vi "WPI_RobotDriveOpen2MotorWithSPARK.vi"(5 "Right Motor Inverted":bool, 7 "Left Motor Inverted":bool, 8 "error in (no error)":errorcluster, 10 "Right Motor":T4=enum."Invalid", 11 "Left Motor":T4=enum."Invalid") -> (0 "error out":errorcluster, 3 "RobotDriveDevRef":T1={"DevStatus"={"status"=FALSE, "code"=0, "source"=""}, "Motors[]"=[], "Square Inputs"=FALSE, "Max Output"=1.0})   [LabVIEW 2025]
doc: "Opens a reference to the robot drive for a two-motor robot using Rev Robotics SPARK motor controllers.\n\nThis software is licensed. Open the labview\\readme\\WPI Robotics Library Open Source License.txt file for more information."
uses:
  <vilib>/Rock Robotics/SystemInterfaces/DIO/FPGA_DIOPWMChannel.ctl
  <vilib>/Rock Robotics/WPI/RobotDrive/WPI_RobotDriveDevRef.ctl
  <vilib>/Rock Robotics/WPI/MotorControl/WPI_MotorControlDeviceRef.ctl
  <vilib>/Rock Robotics/WPI/MotorControl/WPI_MotorControlType.ctl
  <vilib>/Rock Robotics/WPI/PWM/WPI_PWMDeadband.ctl
  <vilib>/Rock Robotics/SystemInterfaces/DIO/FPGA_DIOChannel.ctl
  <vilib>/Rock Robotics/WPI/SafetyOutput/WPI_SafetyOutputConfigMenu.ctl
  <vilib>/Rock Robotics/WPI/MotorControl/WPI_MotorControlOpen SPARK.vi
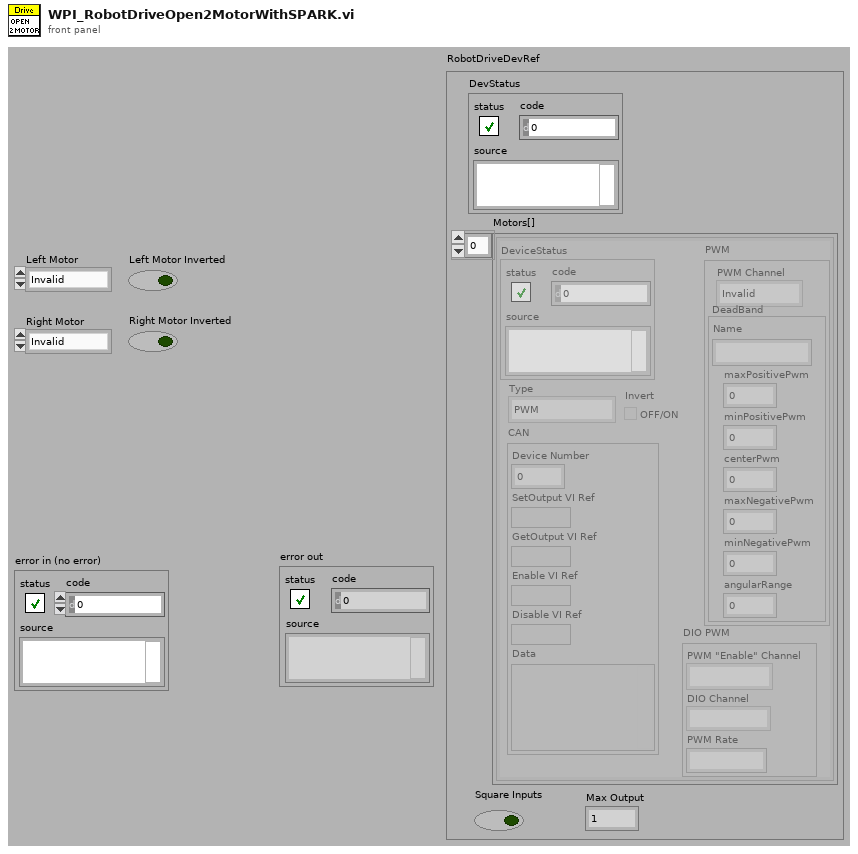
[diagram p1: front panel]
types:
  T1 = typedef "WPI_RobotDriveDevRef.ctl" = cluster{"DevStatus":errorcluster, "Motors[]":T2[], "Square Inputs":bool, "Max Output":dbl}
  T2 = typedef "WPI_MotorControlDeviceRef.ctl" = cluster{"DeviceStatus":errorcluster, "Type":T3, "PWM":cluster{"PWM Channel":T4, "DeadBand":T5}, "CAN":cluster{"Device Number":u8, "SetOutput VI Ref":variant, "GetOutput VI Ref":variant, "Enable VI Ref":variant, "Disable VI Ref":variant, "Data":variant}, "Invert":bool, "DIO PWM":cluster{"PWM \"Enable\" Channel":T4, "DIOChannel":T6, "PWM Rate":dbl}}
  T3 = typedef "WPI_MotorControlType.ctl" = enum16{"PWM", "CAN", "DIO PWM"}
  T4 = typedef "FPGA_DIOPWMChannel.ctl" = enum8{"PWM 0", "PWM 1", "PWM 2", "PWM 3", "PWM 4", "PWM 5", "PWM 6", "PWM 7", "PWM 8", "PWM 9", "PWM MXP 0", "PWM MXP 1", "PWM MXP 2", "PWM MXP 3", "PWM MXP 4", "PWM MXP 5", "PWM MXP 6", "PWM MXP 7", "PWM MXP 8", "PWM MXP 9", "Invalid"}
  T5 = typedef "WPI_PWMDeadband.ctl" = cluster{"Name":string, "maxPositivePwm":i32, "minPositivePwm":i32, "centerPwm":i32, "maxNegativePwm":i32, "minNegativePwm":i32, "angularRange":u16}
  T6 = typedef "FPGA_DIOChannel.ctl" = enum8{"DIO 0", "DIO 1", "DIO 2", "DIO 3", "DIO 4", "DIO 5", "DIO 6", "DIO 7", "DIO 8", "DIO 9", "DIO MXP 0", "DIO MXP 1", "DIO MXP 2", "DIO MXP 3", "DIO MXP 4", "DIO MXP 5", "DIO MXP 6", "DIO MXP 7", "DIO MXP 8", "DIO MXP 9", "DIO MXP 10", "DIO MXP 11", "DIO MXP 12", "DIO MXP 13", "DIO MXP 14", "DIO MXP 15", "SPI Port CS1", "SPI Port CS2", "SPI Port CS3", "SPI Port MISO", "SPI Port MOSI", "Invalid"}
  T7 = typedef "WPI_SafetyOutputConfigMenu.ctl" = enum16{"Enable", "Disable"}
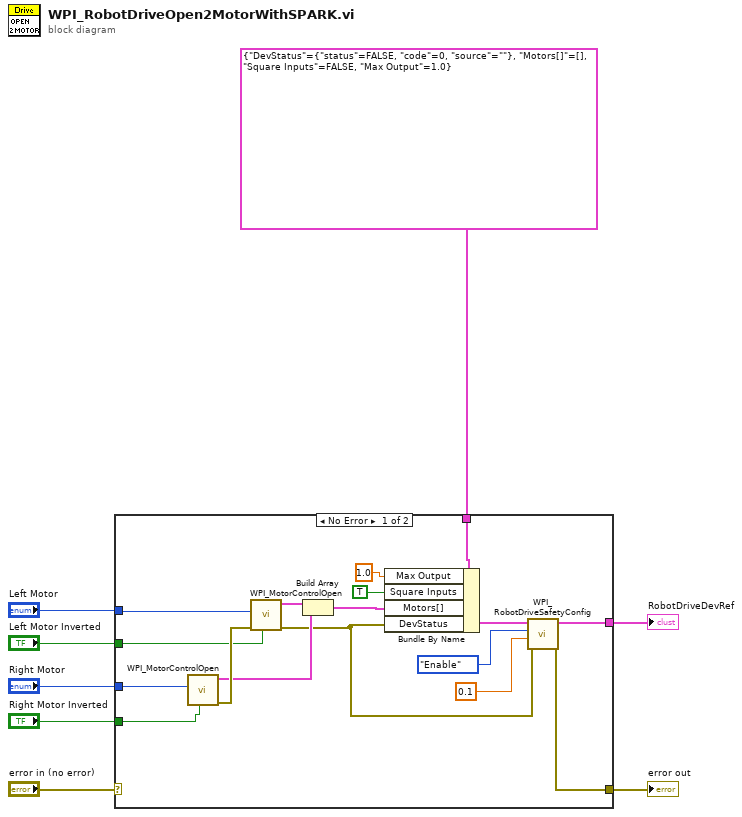
[diagram p0: block diagram]
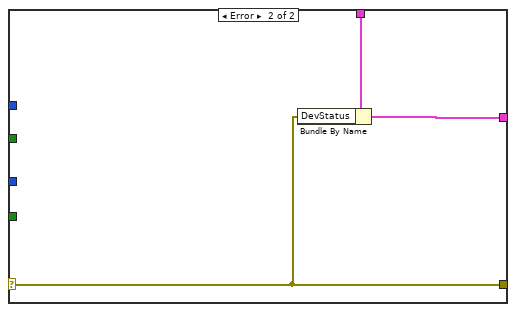
[diagram p2: hidden frame]
diagram:
  n1 = case shown="No Error" "error in (no error)" {
    selector: "error in (no error)" -> [_ w26]
    tunnel: "Left Motor" -> [w23 _]
    tunnel: "Right Motor" -> [w22 _]
    tunnel: [w11 w28] -> w1
    tunnel: "Left Motor Inverted" -> [w17 _]
    tunnel: "Right Motor Inverted" -> [w18 _]
    tunnel: T1 {"DevStatus"={"status"=FALSE, "code"=0, "source"=""}, "Motors[]"=[], "Square Inputs"=FALSE, "Max Output"=1.0} ("RobotDriveDevRef") -> [w24 w27]
    tunnel: [w12 w26] -> w3
    frame No Error {
      n2 = call-poly <vilib>:"WPI_MotorControlOpen.vi"("Invert"=w18, "PWM Channel"=w22) -> ("error out"=w21:errorcluster, "MotorControlDeviceRef"=w19:T2)  [unwired: 2 in, 6 out]
      n3 = call-poly <vilib>:"WPI_MotorControlOpen.vi"("Invert"=w17, "error in (no error)"=w21, "PWM Channel"=w23) -> ("error out"=w13:errorcluster, "MotorControlDeviceRef"=w20:T2)  [unwired: 1 in, 6 out]
      n4 = Build Array(w20, w19) -> (w25:T2[])
      n5 = Bundle By Name(cluster=w24, "Max Output"=1.0, "Square Inputs"=TRUE, "Motors[]"=w25, "DevStatus"=w13) -> (w15:T1)
      n6 = call <vilib>:"WPI_RobotDriveSafetyConfig.vi"("error in (no error)"=w13, "timeout (s)"=0.1, "mode"=WPI_SafetyOutputConfigMenu."Enable", "RobotDriveDevRef"=w15) -> ("error out"=w12:errorcluster, "RobotDriveDevRef"=w11:T1)  [unwired: 6 out]
    }
    frame Error {
      n7 = Bundle By Name(cluster=w27, "DevStatus"=w26) -> (w28:T1)
    }
  }
  "RobotDriveDevRef" <- w1
  "error out" <- w3
